vi "relWaypoint.vi"(7 "Base Point":enum16{"Port", "Midpoint", "Starboard"}(ring), 8 "Error In":errorcluster, 9 "Y coord":dbl, 10 "X coord":dbl, 11 "PassBouy.lvclass":refnum<class "PassBouy.lvclass">) -> (0 "Error Out":errorcluster, 1 "Waypoint Out":refnum<class "Waypoint.lvclass">, 3 "PassBouy.lvclass out":refnum<class "PassBouy.lvclass">)   [LabVIEW 2013]
doc: "This vi takes in an insance of PassBouy class, the distance the waypoint should be along the line formed by the port and starboard bouy (x-coor), the distance the waypoint should be perpendicular to the line formed by the port and starboard bouy (y-coor). Both the x-coor and the y-coor are relative to the Base point which can be the port bouy, the starboard bouy, and the midpoint they form. If the two bouys are at the exact same location this vi will simply output the location of the bouy."
uses:
  PassBouy.lvclass
  Waypoint/Waypoint.lvclass
  Data/TypeDefs/UTM Location.ctl
  <vilib>/Analysis/Matrix/Datatypes/RealMatrix.ctl
  <vilib>/Analysis/baseanly.llb/Unit Vector (DBL).vi
  <vilib>/Analysis/Matrix/Numeric/Conversions/Array To Matrix - RA.vi
  <vilib>/Analysis/Matrix/Numeric/Multiply/Multiply - RM,R.vi
  <vilib>/Analysis/Matrix/Numeric/Conversions/Matrix To Array - RM.vi
  <vilib>/Analysis/Matrix/Numeric/Multiply/Multiply - RM,RM.vi
  <vilib>/Analysis/NI_AALBase.lvlib
  <vilib>/Analysis/Matrix/NI_Matrix.lvlib
panel:
  out "Waypoint Out":T1 {"North" format="%#_10f"; "East" format="%#_8f"}
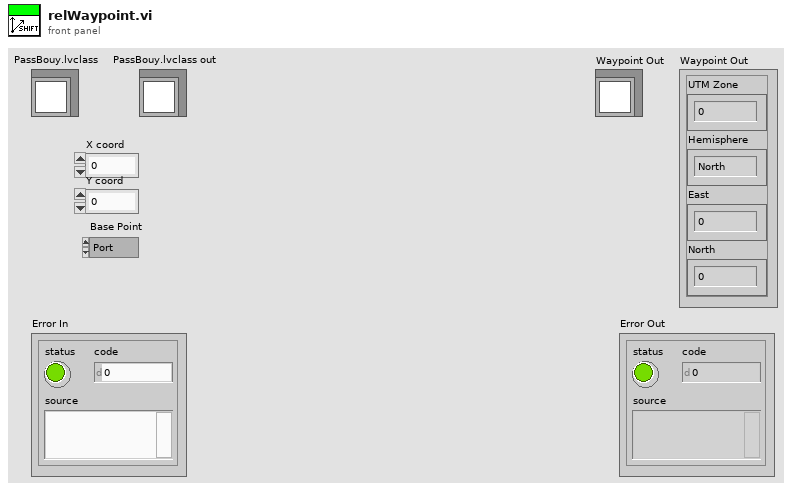
[diagram p1: front panel]
types:
  T1 = typedef "UTM Location.ctl" = cluster{"UTM Zone":dbl, "Hemisphere":enum16{"North", "South"}, "East":dbl, "North":dbl}
  T2 = typedef "NI_Matrix.lvlib/RealMatrix.ctl" = dbl[][]
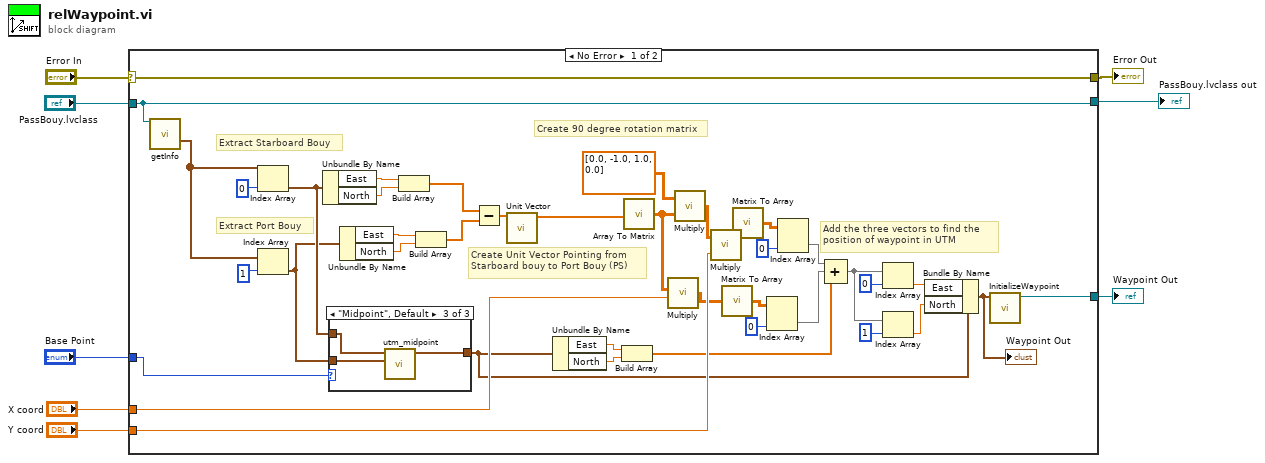
[diagram p0: block diagram]
diagram:
  n1 = case shown="No Error" "Error In" {
    selector: "Error In" -> [w48 w54]
    tunnel: [w48 w54] -> w6
    tunnel: "PassBouy.lvclass" -> [w10 w55]
    tunnel: [w10 w55] -> w7
    tunnel: "X coord" -> [w33 _]
    tunnel: "Y coord" -> [w31 _]
    tunnel: "Base Point" -> [w42 _]
    tunnel: [w18 _] -> w1
    frame No Error {
      # "Add the three vectors to find the \nposition of waypoint in UTM"
      # "Create 90 degree rotation matrix"
      # "Create Unit Vector Pointing from\nStarboard bouy to Port Bouy (PS)"
      # "Extract Port Bouy"
      # "Extract Starboard Bouy"
      n2 = call-dynamic "getInfo.vi"("GenericMission in"=w10) -> ("Points of Interest"=w9:T1[])  [unwired: 6 in, 8 out]
      n3 = Index Array(array=w9, index=0) -> (element=w45:T1)
      n4 = Index Array(array=w9, index=1) -> (element=w39:T1)
      n5 = Unbundle By Name(w45) -> ("East"=w44:dbl, "North"=w43:dbl)
      n6 = case shown="\"Midpoint\", Default" w42 {
        tunnel: w45 -> [w49 _ w53]
        tunnel: w39 -> [_ w50 w52]
        tunnel: [w49 w50 w51] -> w17
        frame "Starboard" {
        }
        frame "Port" {
        }
        frame "Midpoint", Default {
          n7 = call "utm_midpoint.vi"("UTM Location 2"=w52, "UTM Location"=w53) -> ("UTM Location 3"=w51:T1)  [unwired: 7 in, 2 out]
        }
      }
      n8 = Unbundle By Name(w39) -> ("East"=w40:dbl, "North"=w41:dbl)
      n9 = Build Array(w44, w43) -> (w38:dbl[])
      n10 = Build Array(w40, w41) -> (w37:dbl[])
      n11 = Subtract(x=w38, y=w37) -> (x-y=w36:dbl[])
      n12 = call-poly <vilib>:"Unit Vector.vi"("Input Vector"=w36) -> ("Unit Vector"=w35:dbl[])  [unwired: 8 in, 2 out]
      n13 = Unbundle By Name(w17) -> ("East"=w30:dbl, "North"=w29:dbl)
      n14 = Build Array(w30, w29) -> (w24:dbl[])
      n15 = call-poly <vilib>:"Array To Matrix.vi"("Real 1D Array"=w35) -> ("Real Matrix (Column Vector)"=w34:T2)
      n16 = call-poly <vilib>:"Multiply.vi"("Real Scalar c"=w33, "Real Matrix A"=w34) -> ("A * c"=w27:T2)
      n17 = call-poly <vilib>:"Multiply.vi"("Real Matrix B"=w34, "Real Matrix A"=T2 [[0.0, -1.0], [1.0, 0.0]] ("matrix")) -> ("A * B"=w32:T2)
      n18 = call-poly <vilib>:"Multiply.vi"("Real Scalar c"=w31, "Real Matrix A"=w32) -> ("A * c"=w19:T2)
      n19 = call-poly <vilib>:"Matrix To Array.vi"("Real Matrix"=w27) -> ("Real 2D Array"=w26:dbl[][])
      n20 = call-poly <vilib>:"Matrix To Array.vi"("Real Matrix"=w19) -> ("Real 2D Array"=w21:dbl[][])
      n21 = Index Array(array=w26, index (col)=0 ("disabled index (col)")) -> (element=w23:dbl[])  [unwired: 1 in]
      n22 = Index Array(array=w21, index (col)=0 ("disabled index (col)")) -> (element=w20:dbl[])  [unwired: 1 in]
      n23 = Compound Arithmetic op=ADD(w20, w23, w24) -> (w12:dbl[])
      n24 = Index Array(array=w12, index=0) -> (element=w14:dbl)
      n25 = Index Array(array=w12, index=1) -> (element=w11:dbl)
      n26 = Bundle By Name(cluster=w17, "East"=w14, "North"=w11) -> (w16:T1)
      "Waypoint Out" <- w16
      n27 = call "InitializeWaypoint.vi"("Coords"=w16) -> ("Waypoint Out"=w18:refnum<class "Waypoint.lvclass">)  [unwired: 10 in]
    }
    frame Error {
    }
  }
  "Error Out" <- w6
  "PassBouy.lvclass out" <- w7
  "Waypoint Out" <- w1
